vi "Calculate Number of Labels Available to Read (AIM_AIT).vi"(9 "entry count":u32) -> (1 "# of labels available":dbl)   [LabVIEW 2016, in "Ballard Arinc-429 Engine.lvlib"]
uses:
  Ballard Arinc-429 Engine.lvlib
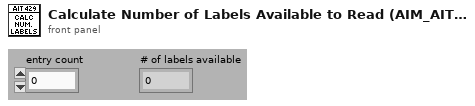
[diagram p1: front panel]
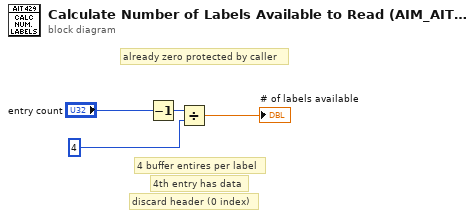
[diagram p0: block diagram]
diagram:
  # "already zero protected by caller"
  # "4 buffer entires per label"
  # "discard header (0 index)"
  # "4th entry has data"
  n1 = Decrement(x="entry count") -> (x-1=w1:u32)
  n2 = Divide(x=w1, y=u32 4 ("x")) -> (x/y=→"# of labels available":dbl)
